vi "Rectangles to Commands.vi"(1 "rects":T4(array[cluster]), 2 "Rectangle Properties":T2(array[cluster])=[{"Speed (um/s)"=2.0, "Direction (For Stroked)"=0, "Start Point"=enum."Bottom Left Corner", "Fill in spacing (um)"=0.3, "Orientation (For Filled)"=enum."Vertical", "Voltage"=0.0}, {"Speed (um/s)"=2.0, "Direction (For Stroked)"=0, "Start Point"=enum."Bottom Left Corner", "Fill in spacing (um)"=0.3, "Orientation (For Filled)"=enum."Vertical", "Voltage"=0.0}, {"Speed (um/s)"=2.0, "Direction (For Stroked)"=0, "Start Point"=enum."Bottom Left Corner", "Fill in spacing (um)"=0.3, "Orientation (For Filled)"=enum."Vertical", "Voltage"=0.0}, {"Speed (um/s)"=2.0, "Direction (For Stroked)"=0, "Start Point"=enum."Bottom Left Corner", "Fill in spacing (um)"=0.3, "Orientation (For Filled)"=enum."Vertical", "Voltage"=0.0}, {"Speed (um/s)"=2.0, "Direction (For Stroked)"=0, "Start Point"=enum."Bottom Left Corner", "Fill in spacing (um)"=0.3, "Orientation (For Filled)"=enum."Vertical", "Voltage"=0.0}, {"Speed (um/s)"=2.0, "Direction (For Stroked)"=0, "Start Point"=enum."Bottom Left Corner", "Fill in spacing (um)"=0.3, "Orientation (For Filled)"=enum."Vertical", "Voltage"=0.0}, {"Speed (um/s)"=2.0, "Direction (For Stroked)"=0, "Start Point"=enum."Bottom Left Corner", "Fill in spacing (um)"=0.3, "Orientation (For Filled)"=enum."Vertical", "Voltage"=0.0}, {"Speed (um/s)"=2.0, "Direction (For Stroked)"=0, "Start Point"=enum."Bottom Left Corner", "Fill in spacing (um)"=0.3, "Orientation (For Filled)"=enum."Vertical", "Voltage"=0.0}, {"Speed (um/s)"=2.0, "Direction (For Stroked)"=0, "Start Point"=enum."Bottom Left Corner", "Fill in spacing (um)"=0.3, "Orientation (For Filled)"=enum."Vertical", "Voltage"=0.0}, {"Speed (um/s)"=2.0, "Direction (For Stroked)"=0, "Start Point"=enum."Bottom Left Corner", "Fill in spacing (um)"=0.3, "Orientation (For Filled)"=enum."Vertical", "Voltage"=0.0}, {"Speed (um/s)"=2.0, "Direction (For Stroked)"=0, "Start Point"=enum."Bottom Left Corner", "Fill in spacing (um)"=0.3, "Orientation (For Filled)"=enum."Vertical", "Voltage"=0.0}, {"Speed (um/s)"=2.0, "Direction (For Stroked)"=0, "Start Point"=enum."Bottom Left Corner", "Fill in spacing (um)"=0.3, "Orientation (For Filled)"=enum."Vertical", "Voltage"=0.0}, {"Speed (um/s)"=2.0, "Direction (For Stroked)"=0, "Start Point"=enum."Bottom Left Corner", "Fill in spacing (um)"=0.3, "Orientation (For Filled)"=enum."Vertical", "Voltage"=0.0}, {"Speed (um/s)"=2.0, "Direction (For Stroked)"=0, "Start Point"=enum."Bottom Left Corner", "Fill in spacing (um)"=0.3, "Orientation (For Filled)"=enum."Vertical", "Voltage"=0.0}, {"Speed (um/s)"=2.0, "Direction (For Stroked)"=0, "Start Point"=enum."Bottom Left Corner", "Fill in spacing (um)"=0.3, "Orientation (For Filled)"=enum."Vertical", "Voltage"=0.0}, {"Speed (um/s)"=2.0, "Direction (For Stroked)"=0, "Start Point"=enum."Bottom Left Corner", "Fill in spacing (um)"=0.3, "Orientation (For Filled)"=enum."Vertical", "Voltage"=0.0}, {"Speed (um/s)"=2.0, "Direction (For Stroked)"=0, "Start Point"=enum."Bottom Left Corner", "Fill in spacing (um)"=0.3, "Orientation (For Filled)"=enum."Vertical", "Voltage"=0.0}, {"Speed (um/s)"=2.0, "Direction (For Stroked)"=0, "Start Point"=enum."Bottom Left Corner", "Fill in spacing (um)"=0.3, "Orientation (For Filled)"=enum."Vertical", "Voltage"=0.0}, {"Speed (um/s)"=2.0, "Direction (For Stroked)"=0, "Start Point"=enum."Bottom Left Corner", "Fill in spacing (um)"=0.3, "Orientation (For Filled)"=enum."Vertical", "Voltage"=0.0}, {"Speed (um/s)"=2.0, "Direction (For Stroked)"=0, "Start Point"=enum."Bottom Left Corner", "Fill in spacing (um)"=0.3, "Orientation (For Filled)"=enum."Vertical", "Voltage"=0.0}, {"Speed (um/s)"=2.0, "Direction (For Stroked)"=0, "Start Point"=enum."Bottom Left Corner", "Fill in spacing (um)"=0.3, "Orientation (For Filled)"=enum."Vertical", "Voltage"=0.0}, {"Speed (um/s)"=2.0, "Direction (For Stroked)"=0, "Start Point"=enum."Bottom Left Corner", "Fill in spacing (um)"=0.3, "Orientation (For Filled)"=enum."Vertical", "Voltage"=0.0}, {"Speed (um/s)"=2.0, "Direction (For Stroked)"=0, "Start Point"=enum."Bottom Left Corner", "Fill in spacing (um)"=0.3, "Orientation (For Filled)"=enum."Vertical", "Voltage"=0.0}, {"Speed (um/s)"=2.0, "Direction (For Stroked)"=0, "Start Point"=enum."Bottom Left Corner", "Fill in spacing (um)"=0.3, "Orientation (For Filled)"=enum."Vertical", "Voltage"=0.0}, {"Speed (um/s)"=2.0, "Direction (For Stroked)"=0, "Start Point"=enum."Bottom Left Corner", "Fill in spacing (um)"=0.3, "Orientation (For Filled)"=enum."Vertical", "Voltage"=0.0}, {"Speed (um/s)"=2.0, "Direction (For Stroked)"=0, "Start Point"=enum."Bottom Left Corner", "Fill in spacing (um)"=0.3, "Orientation (For Filled)"=enum."Vertical", "Voltage"=0.0}, {"Speed (um/s)"=2.0, "Direction (For Stroked)"=0, "Start Point"=enum."Bottom Left Corner", "Fill in spacing (um)"=0.3, "Orientation (For Filled)"=enum."Vertical", "Voltage"=0.0}, {"Speed (um/s)"=2.0, "Direction (For Stroked)"=0, "Start Point"=enum."Bottom Left Corner", "Fill in spacing (um)"=0.3, "Orientation (For Filled)"=enum."Vertical", "Voltage"=0.0}, {"Speed (um/s)"=2.0, "Direction (For Stroked)"=0, "Start Point"=enum."Bottom Left Corner", "Fill in spacing (um)"=0.3, "Orientation (For Filled)"=enum."Vertical", "Voltage"=0.0}, {"Speed (um/s)"=2.0, "Direction (For Stroked)"=0, "Start Point"=enum."Bottom Left Corner", "Fill in spacing (um)"=0.3, "Orientation (For Filled)"=enum."Vertical", "Voltage"=0.0}] {"Direction (For Stroked)" items=["Clockwise", "Counterclockwise"]}) -> (0 "Lithography information":T1(array[cluster]))   [LabVIEW 2013]
doc: "This VI processes the rectangles' data and outputs lithography data."
uses:
  <vilib>/Analysis/Matrix/Datatypes/RealMatrix.ctl
  <vilib>/Levylab/General AFM Lithography/subvi/simulator/Global Variables.vi
  <vilib>/Analysis/Matrix/NI_Matrix.lvlib
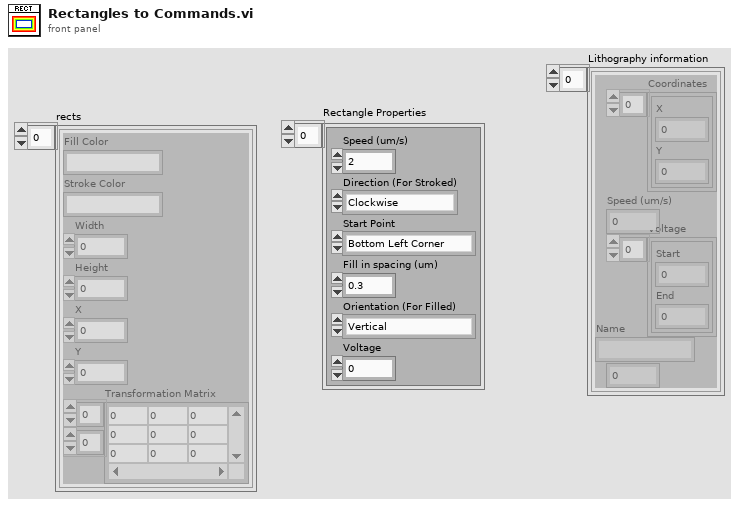
[diagram p1: front panel]
types:
  T1 = cluster{"Coordinates":cluster{"X":dbl, "Y":dbl}[], "Speed (um/s)":dbl, "Voltage":cluster{"Start":dbl, "End":dbl}[], "Name":string, "Order":i32}[]
  T2 = cluster{"Speed (um/s)":dbl, "Direction (For Stroked)":u16, "Start Point":enum16{"Bottom Left Corner", "Bottom Right Corner", "Top Left Corner", "Top Right Corner"}, "Fill in spacing (um)":dbl, "Orientation (For Filled)":enum16{"Horizontal", "Vertical"}, "Voltage":dbl}[]
  T3 = typedef "NI_Matrix.lvlib/RealMatrix.ctl" = dbl[][]
  T4 = cluster{"Fill Color":string, "Stroke Color":string, "Width":dbl, "Height":dbl, "X":dbl, "Y":dbl, "Transformation Matrix":T3}[]
  T5 = enum16{"Bottom Left Corner", "Bottom Right Corner", "Top Left Corner", "Top Right Corner"}
  T6 = cluster{cluster{"X":dbl, "Y":dbl}[], "Speed (um/s)":dbl, cluster{"Voltage":dbl, "Voltage":dbl}[], string, i32}
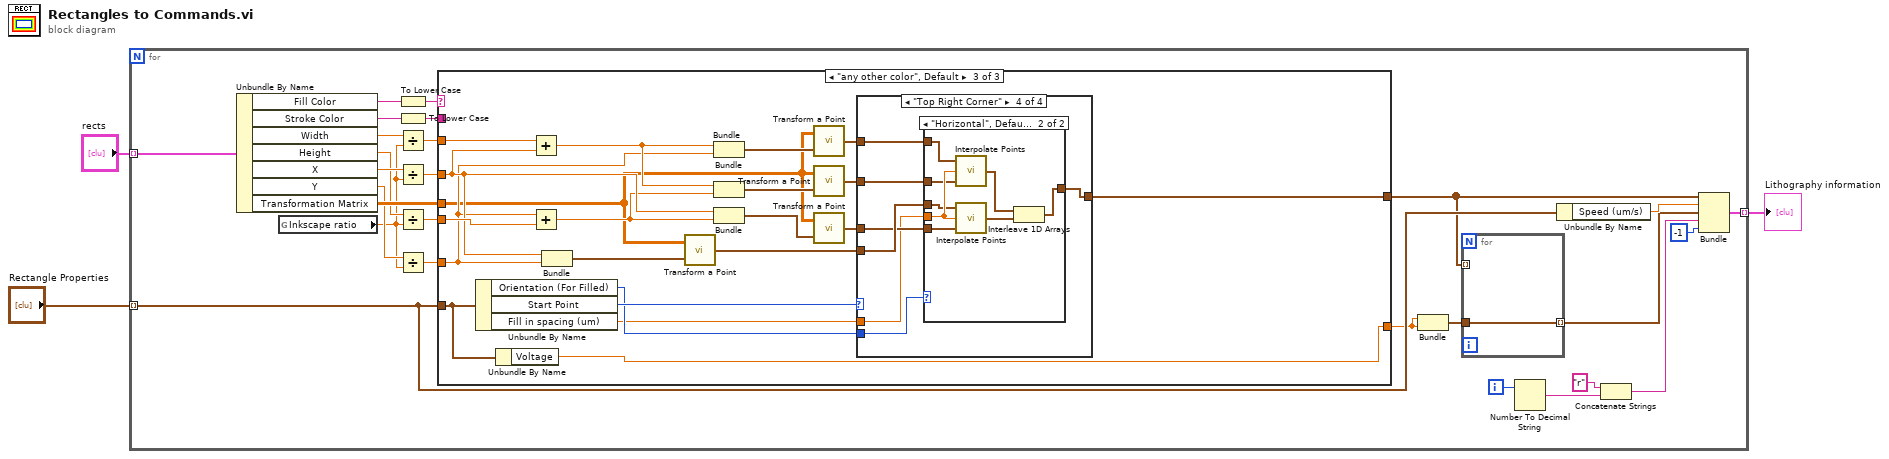
[diagram p0: block diagram]
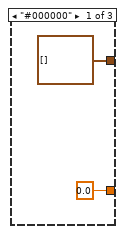
[diagram p2: hidden frame]
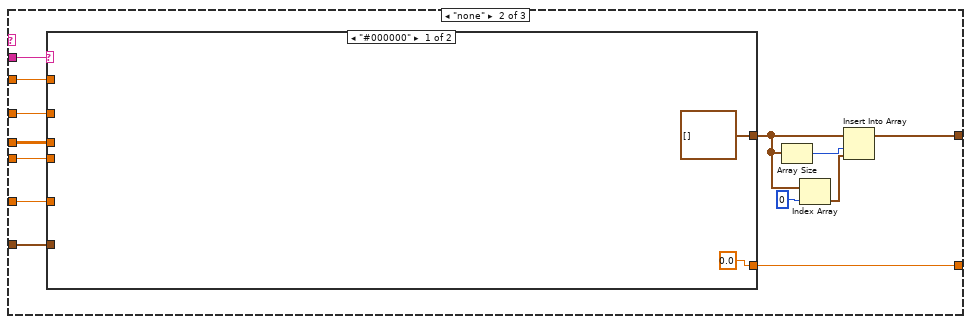
[diagram p3: hidden frame]
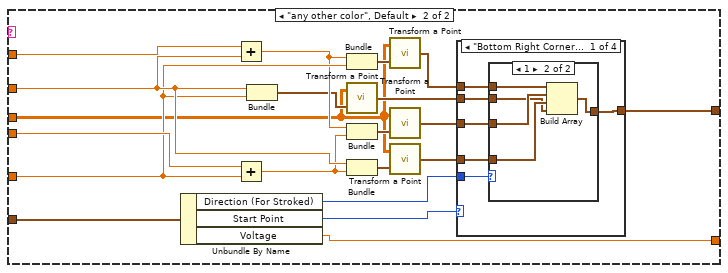
[diagram p4: hidden frame]
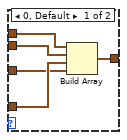
[diagram p5: hidden frame]
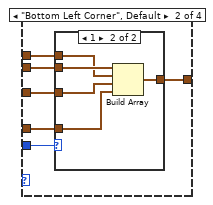
[diagram p6: hidden frame]
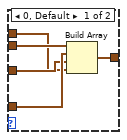
[diagram p7: hidden frame]
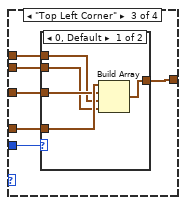
[diagram p8: hidden frame]
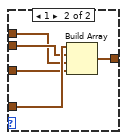
[diagram p9: hidden frame]
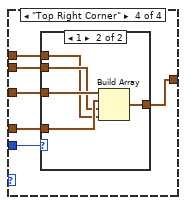
[diagram p10: hidden frame]
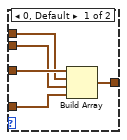
[diagram p11: hidden frame]
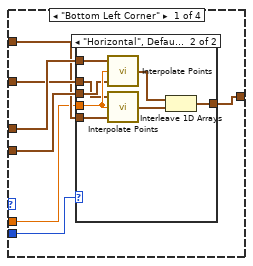
[diagram p12: hidden frame]
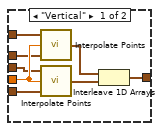
[diagram p13: hidden frame]
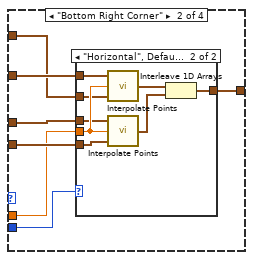
[diagram p14: hidden frame]
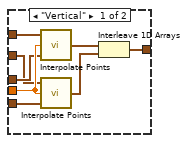
[diagram p15: hidden frame]
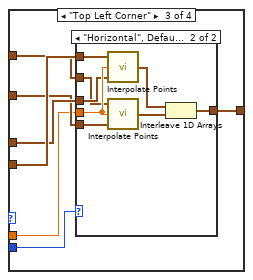
[diagram p16: hidden frame]
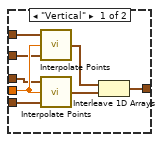
[diagram p17: hidden frame]
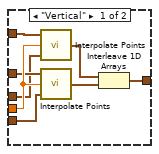
[diagram p18: hidden frame]
diagram:
  n1 = for {
    tunnel: "rects" -> [w30] mode=indexing
    tunnel: "Rectangle Properties" -> [w24] mode=indexing
    tunnel: [w25] -> w1 mode=indexing
    i -> [w21]
    n2 = Unbundle By Name(w30) -> ("Fill Color"=w29:string, "Stroke Color"=w27:string, "Width"=w16:dbl, "Height"=w10:dbl, "X"=w14:dbl, "Y"=w12:dbl, "Transformation Matrix"=w18:T3)
    n3 = global read "Global Variables.vi" "Inkscape ratio"() -> (w8:dbl)
    n4 = To Lower Case(string=w29) -> (all lower case string=w28:string)
    n5 = To Lower Case(string=w27) -> (all lower case string=w26:string)
    n6 = Divide(x=w16, y=w8) -> (x/y=w15:dbl)
    n7 = Divide(x=w14, y=w8) -> (x/y=w13:dbl)
    n8 = Divide(x=w10, y=w8) -> (x/y=w9:dbl)
    n9 = Divide(x=w12, y=w8) -> (x/y=w11:dbl)
    n10 = case shown="\"any other color\", Default" w28 {
      tunnel: w26 -> [_ w42 _]
      tunnel: w15 -> [_ w46 w150]
      tunnel: w9 -> [_ w45 w149]
      tunnel: w13 -> [_ w44 w148]
      tunnel: w11 -> [_ w43 w145]
      tunnel: w24 -> [_ w35 w134]
      tunnel: [cluster{"X":dbl, "Y":dbl}[] [] w37 w153] -> w7
      tunnel: w18 -> [_ w36 w135]
      tunnel: [0.0 ("End Voltage") w34 w133] -> w5
      frame "#000000" {
      }
      frame "none" {
        n11 = case shown="\"#000000\"" w42 {
          tunnel: w46 -> [_ w67]
          tunnel: w45 -> [_ w68]
          tunnel: w44 -> [_ w66]
          tunnel: w43 -> [_ w64]
          tunnel: [cluster{"X":dbl, "Y":dbl}[] [] w59] -> w38
          tunnel: w35 -> [_ w62]
          tunnel: w36 -> [_ w50]
          tunnel: [0.0 ("Voltage") w49] -> w34
          frame "#000000" {
          }
          frame "any other color", Default {
            n12 = Unbundle By Name(w62) -> ("Direction (For Stroked)"=w60:u16, "Start Point"=w61:T5, "Voltage"=w49:dbl)
            n13 = Add(x=w67, y=w66) -> (x+y=w63:dbl)
            n14 = Add(x=w68, y=w64) -> (x+y=w65:dbl)
            n15 = Bundle(w66, w64) -> (w56:cluster{dbl, dbl})  [unwired: 1 in]
            n16 = Bundle(w63, w64) -> (w51:cluster{dbl, dbl})  [unwired: 1 in]
            n17 = call <vilib>:"Transform a Point.vi"("Point to Transform"=w56, "Transformation Matrix"=w50) -> ("Transformed Point"=w55:cluster{"X":dbl, "Y":dbl})
            n18 = Bundle(w63, w65) -> (w53:cluster{dbl, dbl})  [unwired: 1 in]
            n19 = Bundle(w66, w65) -> (w58:cluster{dbl, dbl})  [unwired: 1 in]
            n20 = call <vilib>:"Transform a Point.vi"("Point to Transform"=w51, "Transformation Matrix"=w50) -> ("Transformed Point"=w52:cluster{"X":dbl, "Y":dbl})
            n21 = call <vilib>:"Transform a Point.vi"("Point to Transform"=w53, "Transformation Matrix"=w50) -> ("Transformed Point"=w54:cluster{"X":dbl, "Y":dbl})
            n22 = call <vilib>:"Transform a Point.vi"("Point to Transform"=w58, "Transformation Matrix"=w50) -> ("Transformed Point"=w57:cluster{"X":dbl, "Y":dbl})
            n23 = case shown="\"Bottom Right Corner\"" w61 {
              tunnel: w60 -> [w74 w90 w106 w122]
              tunnel: [w73 w89 w105 w121] -> w59
              tunnel: w55 -> [w71 w88 w101 w118]
              tunnel: w57 -> [w70 w87 w104 w117]
              tunnel: w54 -> [w69 w86 w103 w120]
              tunnel: w52 -> [w72 w85 w102 w119]
              frame "Bottom Right Corner" {
                n24 = case shown="1" w74 {
                  tunnel: [w79 w84] -> w73
                  tunnel: w72 -> [w78 w83]
                  tunnel: w71 -> [w77 w80]
                  tunnel: w70 -> [w76 w81]
                  tunnel: w69 -> [w75 w82]
                  frame 0, Default {
                    n25 = Build Array(w78, w77, w76, w75) -> (w79:cluster{"X":dbl, "Y":dbl}[])
                  }
                  frame 1 {
                    n26 = Build Array(w83, w82, w81, w80) -> (w84:cluster{"X":dbl, "Y":dbl}[])
                  }
                }
              }
              frame "Bottom Left Corner", Default {
                n27 = case shown="1" w90 {
                  tunnel: [w95 w100] -> w89
                  tunnel: w88 -> [w94 w99]
                  tunnel: w87 -> [w93 w96]
                  tunnel: w86 -> [w92 w97]
                  tunnel: w85 -> [w91 w98]
                  frame 0, Default {
                    n28 = Build Array(w94, w93, w92, w91) -> (w95:cluster{"X":dbl, "Y":dbl}[])
                  }
                  frame 1 {
                    n29 = Build Array(w99, w98, w97, w96) -> (w100:cluster{"X":dbl, "Y":dbl}[])
                  }
                }
              }
              frame "Top Left Corner" {
                n30 = case shown="0, Default" w106 {
                  tunnel: [w111 w116] -> w105
                  tunnel: w104 -> [w110 w115]
                  tunnel: w103 -> [w109 w112]
                  tunnel: w102 -> [w108 w113]
                  tunnel: w101 -> [w107 w114]
                  frame 0, Default {
                    n31 = Build Array(w110, w109, w108, w107) -> (w111:cluster{"X":dbl, "Y":dbl}[])
                  }
                  frame 1 {
                    n32 = Build Array(w115, w114, w113, w112) -> (w116:cluster{"X":dbl, "Y":dbl}[])
                  }
                }
              }
              frame "Top Right Corner" {
                n33 = case shown="1" w122 {
                  tunnel: [w127 w132] -> w121
                  tunnel: w120 -> [w126 w131]
                  tunnel: w119 -> [w125 w128]
                  tunnel: w118 -> [w124 w129]
                  tunnel: w117 -> [w123 w130]
                  frame 0, Default {
                    n34 = Build Array(w126, w125, w124, w123) -> (w127:cluster{"X":dbl, "Y":dbl}[])
                  }
                  frame 1 {
                    n35 = Build Array(w131, w130, w129, w128) -> (w132:cluster{"X":dbl, "Y":dbl}[])
                  }
                }
              }
            }
          }
        }
        n36 = Array Size(array=w38) -> (size(s)=w41:i32)
        n37 = Index Array(array=w38, index=0) -> (element=w40:cluster{"X":dbl, "Y":dbl})
        n38 = Insert Into Array(array=w38, index=w41, new element=w40) -> (w37:cluster{"X":dbl, "Y":dbl}[])
      }
      frame "any other color", Default {
        n39 = Unbundle By Name(w134) -> ("Orientation (For Filled)"=w151:enum16{"Horizontal", "Vertical"}, "Start Point"=w152:T5, "Fill in spacing (um)"=w144:dbl)
        n40 = Unbundle By Name(w134) -> ("Voltage"=w133:dbl)
        n41 = Add(x=w150, y=w148) -> (x+y=w146:dbl)
        n42 = Add(x=w145, y=w149) -> (x+y=w147:dbl)
        n43 = Bundle(w148, w145) -> (w143:cluster{dbl, dbl})  [unwired: 1 in]
        n44 = call <vilib>:"Transform a Point.vi"("Point to Transform"=w143, "Transformation Matrix"=w135) -> ("Transformed Point"=w142:cluster{"X":dbl, "Y":dbl})
        n45 = Bundle(w146, w145) -> (w136:cluster{dbl, dbl})  [unwired: 1 in]
        n46 = Bundle(w146, w147) -> (w141:cluster{dbl, dbl})  [unwired: 1 in]
        n47 = Bundle(w148, w147) -> (w139:cluster{dbl, dbl})  [unwired: 1 in]
        n48 = call <vilib>:"Transform a Point.vi"("Point to Transform"=w136, "Transformation Matrix"=w135) -> ("Transformed Point"=w137:cluster{"X":dbl, "Y":dbl})
        n49 = call <vilib>:"Transform a Point.vi"("Point to Transform"=w141, "Transformation Matrix"=w135) -> ("Transformed Point"=w140:cluster{"X":dbl, "Y":dbl})
        n50 = call <vilib>:"Transform a Point.vi"("Point to Transform"=w139, "Transformation Matrix"=w135) -> ("Transformed Point"=w138:cluster{"X":dbl, "Y":dbl})
        n51 = case shown="\"Top Right Corner\"" w152 {
          tunnel: w151 -> [w160 w183 w206 w229]
          tunnel: [w159 w182 w205 w228] -> w153
          tunnel: w137 -> [w155 w178 w201 w224]
          tunnel: w140 -> [w156 w179 w202 w225]
          tunnel: w138 -> [w157 w180 w203 w226]
          tunnel: w142 -> [w158 w181 w204 w227]
          tunnel: w144 -> [w154 w177 w200 w223]
          frame "Bottom Left Corner" {
            n52 = case shown="\"Horizontal\", Default" w160 {
              tunnel: [w166 w176] -> w159
              tunnel: w158 -> [w164 w171]
              tunnel: w157 -> [w162 w172]
              tunnel: w156 -> [w161 w170]
              tunnel: w155 -> [w163 w169]
              tunnel: w154 -> [w165 w175]
              frame "Vertical" {
                n53 = call <vilib>:"Interpolate Points.vi"("End Point"=w161, "Distance between Points"=w165, "Start Point"=w162) -> ("Output Point Array"=w168:cluster{"X":dbl, "Y":dbl}[])
                n54 = call <vilib>:"Interpolate Points.vi"("End Point"=w163, "Distance between Points"=w165, "Start Point"=w164) -> ("Output Point Array"=w167:cluster{"X":dbl, "Y":dbl}[])
                n55 = Interleave 1D Arrays(w168, w167) -> (w166:cluster{"X":dbl, "Y":dbl}[])
              }
              frame "Horizontal", Default {
                n56 = call <vilib>:"Interpolate Points.vi"("End Point"=w171, "Distance between Points"=w175, "Start Point"=w172) -> ("Output Point Array"=w174:cluster{"X":dbl, "Y":dbl}[])
                n57 = call <vilib>:"Interpolate Points.vi"("End Point"=w169, "Distance between Points"=w175, "Start Point"=w170) -> ("Output Point Array"=w173:cluster{"X":dbl, "Y":dbl}[])
                n58 = Interleave 1D Arrays(w174, w173) -> (w176:cluster{"X":dbl, "Y":dbl}[])
              }
            }
          }
          frame "Bottom Right Corner" {
            n59 = case shown="\"Horizontal\", Default" w183 {
              tunnel: [w189 w199] -> w182
              tunnel: w181 -> [w184 w193]
              tunnel: w180 -> [w186 w192]
              tunnel: w179 -> [w187 w195]
              tunnel: w178 -> [w185 w194]
              tunnel: w177 -> [w188 w198]
              frame "Vertical" {
                n60 = call <vilib>:"Interpolate Points.vi"("End Point"=w186, "Distance between Points"=w188, "Start Point"=w187) -> ("Output Point Array"=w191:cluster{"X":dbl, "Y":dbl}[])
                n61 = call <vilib>:"Interpolate Points.vi"("End Point"=w184, "Distance between Points"=w188, "Start Point"=w185) -> ("Output Point Array"=w190:cluster{"X":dbl, "Y":dbl}[])
                n62 = Interleave 1D Arrays(w191, w190) -> (w189:cluster{"X":dbl, "Y":dbl}[])
              }
              frame "Horizontal", Default {
                n63 = call <vilib>:"Interpolate Points.vi"("End Point"=w194, "Distance between Points"=w198, "Start Point"=w195) -> ("Output Point Array"=w197:cluster{"X":dbl, "Y":dbl}[])
                n64 = call <vilib>:"Interpolate Points.vi"("End Point"=w193, "Distance between Points"=w198, "Start Point"=w192) -> ("Output Point Array"=w196:cluster{"X":dbl, "Y":dbl}[])
                n65 = Interleave 1D Arrays(w197, w196) -> (w199:cluster{"X":dbl, "Y":dbl}[])
              }
            }
          }
          frame "Top Left Corner" {
            n66 = case shown="\"Horizontal\", Default" w206 {
              tunnel: [w212 w222] -> w205
              tunnel: w204 -> [w210 w218]
              tunnel: w203 -> [w208 w217]
              tunnel: w202 -> [w207 w215]
              tunnel: w201 -> [w209 w216]
              tunnel: w200 -> [w211 w221]
              frame "Vertical" {
                n67 = call <vilib>:"Interpolate Points.vi"("End Point"=w209, "Distance between Points"=w211, "Start Point"=w210) -> ("Output Point Array"=w214:cluster{"X":dbl, "Y":dbl}[])
                n68 = call <vilib>:"Interpolate Points.vi"("End Point"=w207, "Distance between Points"=w211, "Start Point"=w208) -> ("Output Point Array"=w213:cluster{"X":dbl, "Y":dbl}[])
                n69 = Interleave 1D Arrays(w214, w213) -> (w212:cluster{"X":dbl, "Y":dbl}[])
              }
              frame "Horizontal", Default {
                n70 = call <vilib>:"Interpolate Points.vi"("End Point"=w217, "Distance between Points"=w221, "Start Point"=w218) -> ("Output Point Array"=w220:cluster{"X":dbl, "Y":dbl}[])
                n71 = call <vilib>:"Interpolate Points.vi"("End Point"=w215, "Distance between Points"=w221, "Start Point"=w216) -> ("Output Point Array"=w219:cluster{"X":dbl, "Y":dbl}[])
                n72 = Interleave 1D Arrays(w220, w219) -> (w222:cluster{"X":dbl, "Y":dbl}[])
              }
            }
          }
          frame "Top Right Corner" {
            n73 = case shown="\"Horizontal\", Default" w229 {
              tunnel: [w235 w245] -> w228
              tunnel: w227 -> [w230 w239]
              tunnel: w226 -> [w232 w238]
              tunnel: w225 -> [w233 w240]
              tunnel: w224 -> [w231 w241]
              tunnel: w223 -> [w234 w244]
              frame "Vertical" {
                n74 = call <vilib>:"Interpolate Points.vi"("End Point"=w230, "Distance between Points"=w234, "Start Point"=w231) -> ("Output Point Array"=w237:cluster{"X":dbl, "Y":dbl}[])
                n75 = call <vilib>:"Interpolate Points.vi"("End Point"=w232, "Distance between Points"=w234, "Start Point"=w233) -> ("Output Point Array"=w236:cluster{"X":dbl, "Y":dbl}[])
                n76 = Interleave 1D Arrays(w237, w236) -> (w235:cluster{"X":dbl, "Y":dbl}[])
              }
              frame "Horizontal", Default {
                n77 = call <vilib>:"Interpolate Points.vi"("End Point"=w240, "Distance between Points"=w244, "Start Point"=w241) -> ("Output Point Array"=w243:cluster{"X":dbl, "Y":dbl}[])
                n78 = call <vilib>:"Interpolate Points.vi"("End Point"=w238, "Distance between Points"=w244, "Start Point"=w239) -> ("Output Point Array"=w242:cluster{"X":dbl, "Y":dbl}[])
                n79 = Interleave 1D Arrays(w243, w242) -> (w245:cluster{"X":dbl, "Y":dbl}[])
              }
            }
          }
        }
      }
    }
    n80 = Bundle("Voltage"=w5, "Voltage"=w5) -> (w4:cluster{"Voltage":dbl, "Voltage":dbl})  [unwired: 1 in]
    n81 = for {
      tunnel: w7 -> [_] mode=indexing
      tunnel: w4 -> [w31]
      tunnel: [w31] -> w6 mode=indexing
    }
    n82 = Number To Decimal String(number=w21) -> (decimal integer string=w20:string)  [unwired: 1 in]
    n83 = Unbundle By Name(w24) -> ("Speed (um/s)"=w23:dbl)
    n84 = Concatenate Strings("r", w20) -> (w19:string)
    n85 = Bundle(w7, "Speed (um/s)"=w23, w6, w19, -1) -> (w25:T6)  [unwired: 1 in]
  }
  "Lithography information" <- w1
